vi "Read room1.vi"(8 "error in (no error)":errorcluster, 11 "Door in":refnum<class "Door.lvclass">) -> (0 "error out":errorcluster, 2 "room1":refnum<data-value>, 3 "Door out":refnum<class "Door.lvclass">)   [LabVIEW 2016, in "Door.lvclass"]
uses:
  Door.lvclass
  Room/Room.lvclass
  Door.lvclass/Door.ctl
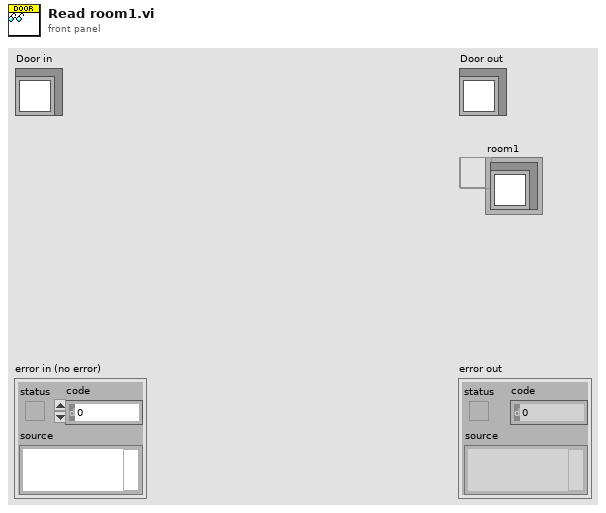
[diagram p1: front panel]
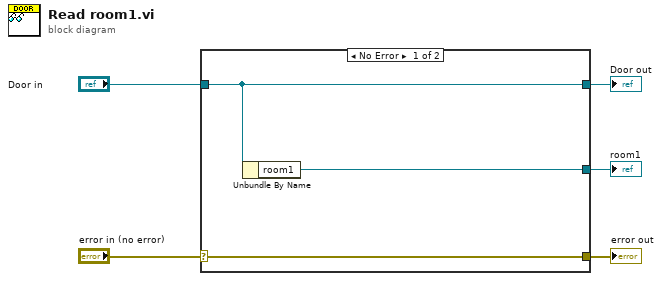
[diagram p0: block diagram]
diagram:
  n1 = case shown="No Error" "error in (no error)" {
    selector: "error in (no error)" -> [w8 w9]
    tunnel: [w8 w9] -> w4
    tunnel: [w7 w10] -> w2
    tunnel: "Door in" -> [w7 w10]
    tunnel: [w6 _] -> w1
    frame No Error {
      n2 = Unbundle By Name(w7) -> ("room1"=w6:refnum<data-value>)
    }
    frame Error {
    }
  }
  "error out" <- w4
  "Door out" <- w2
  "room1" <- w1
